vi "Camera dynamic image streaming.vi"(10 "Camera label indexing":u32[](array[numeric]), 11 "Images_Array_in":T1[](array[typedef])) -> (2 "Display array":bool[](array[boolean]), 3 "Output image array":T1[](array[typedef]))   [LabVIEW 2015]
uses:
  <vilib>/vision/Image Controls.llb/IMAQ Image.ctl
panel:
  in  "Number of racks":u8
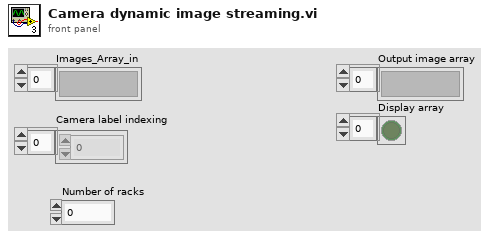
[diagram p1: front panel]
types:
  T1 = typedef "IMAQ Image.ctl" = refnum<image>
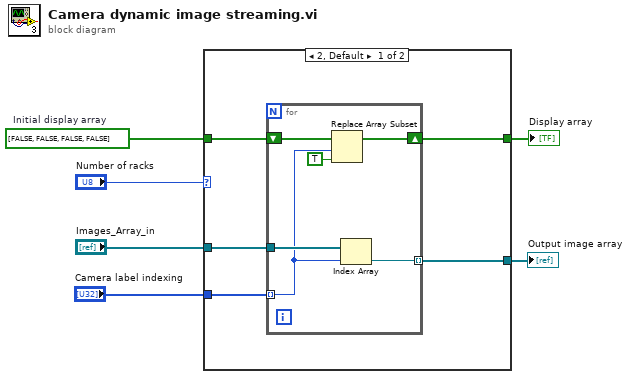
[diagram p0: block diagram]
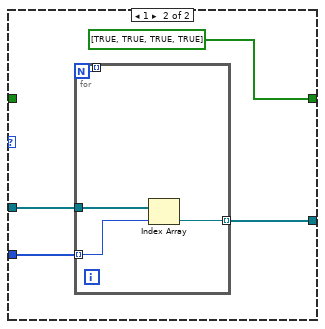
[diagram p2: hidden frame]
diagram:
  w2 = bool[] [FALSE, FALSE, FALSE, FALSE]  # Initial display array
  n1 = case shown="2, Default" "Number of racks" {
    tunnel: "Images_Array_in" -> [w9 w21]
    tunnel: "Camera label indexing" -> [w8 w20]
    tunnel: [w7 w19] -> w4
    tunnel: w2 -> [w11 _]
    tunnel: [w10 bool[] [TRUE, TRUE, TRUE, TRUE] ("Initial display array")] -> w1
    frame 2, Default {
      n2 = for {
        tunnel: w9 -> [w17]
        tunnel: w8 -> [w14] mode=indexing
        tunnel: [w16] -> w7 mode=indexing
        shift-right: [w12] -> w10
        shift-left: w11 -> [w15]
        n3 = Replace Array Subset(array=w15, new element=TRUE ("new element/subarray"), index=w14) -> (w12:bool[])
        n4 = Index Array(array=w17, index=w14) -> (element=w16:T1)
      }
    }
    frame 1 {
      n5 = for {
        N -> [w22]
        tunnel: w21 -> [w25]
        tunnel: w20 -> [w23] mode=indexing
        tunnel: [w24] -> w19 mode=indexing
        tunnel: [w22] -> _ mode=indexing
        n6 = Index Array(array=w25, index=w23) -> (element=w24:T1)
      }
    }
  }
  "Output image array" <- w4
  "Display array" <- w1
